vi "OCV Clear Acquisition.vi"(8 "error in (no error)":errorcluster, 11 "Refnum in":refnum<k21>) -> (0 "error out":errorcluster, 4 "Clear Time (ms)":u32=46)   [LabVIEW 2019]
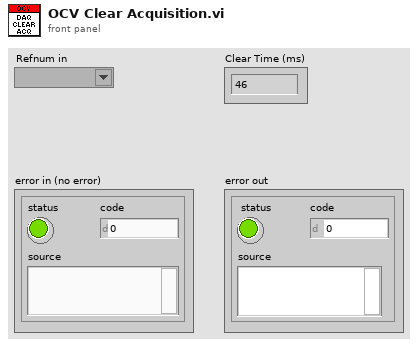
[diagram p1: front panel]
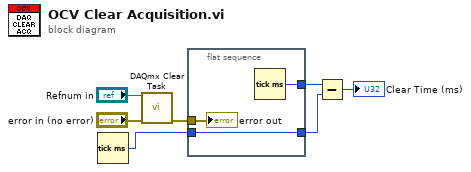
[diagram p0: block diagram]
diagram:
  n1 = Tick Count (ms)() -> (millisecond timer value=w1:u32)
  n2 = call <vilib>:"DAQmx Clear Task.vi"("task in"="Refnum in", "error in"="error in (no error)") -> ("error out"=w6:errorcluster)  [unwired: 13 in]
  n3 = flat-sequence {
    tunnel: w6 -> [w9]
    tunnel: [w10] -> w3
    tunnel: w1 -> [w8]
    tunnel: [w8] -> w4
    frame #0 {
      n4 = Tick Count (ms)() -> (millisecond timer value=w10:u32)
      "error out" <- w9
    }
  }
  n5 = Subtract(x=w3, y=w4) -> (x-y=→"Clear Time (ms)":u32)
